vi "Resistance to temp.vi"(11 "Resistance":dbl format="%#_13p") -> (3 "Temperature":dbl)   [LabVIEW 2021]
uses:
  controls/comparison selection.ctl
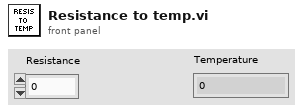
[diagram p1: front panel]
types:
  T1 = typedef "comparison selection.ctl" = enum16{"None", "in-range?", "less than?", "greater than?", "equal to?", "not equal to?", "less or equal to?", "greater or equal to?"}
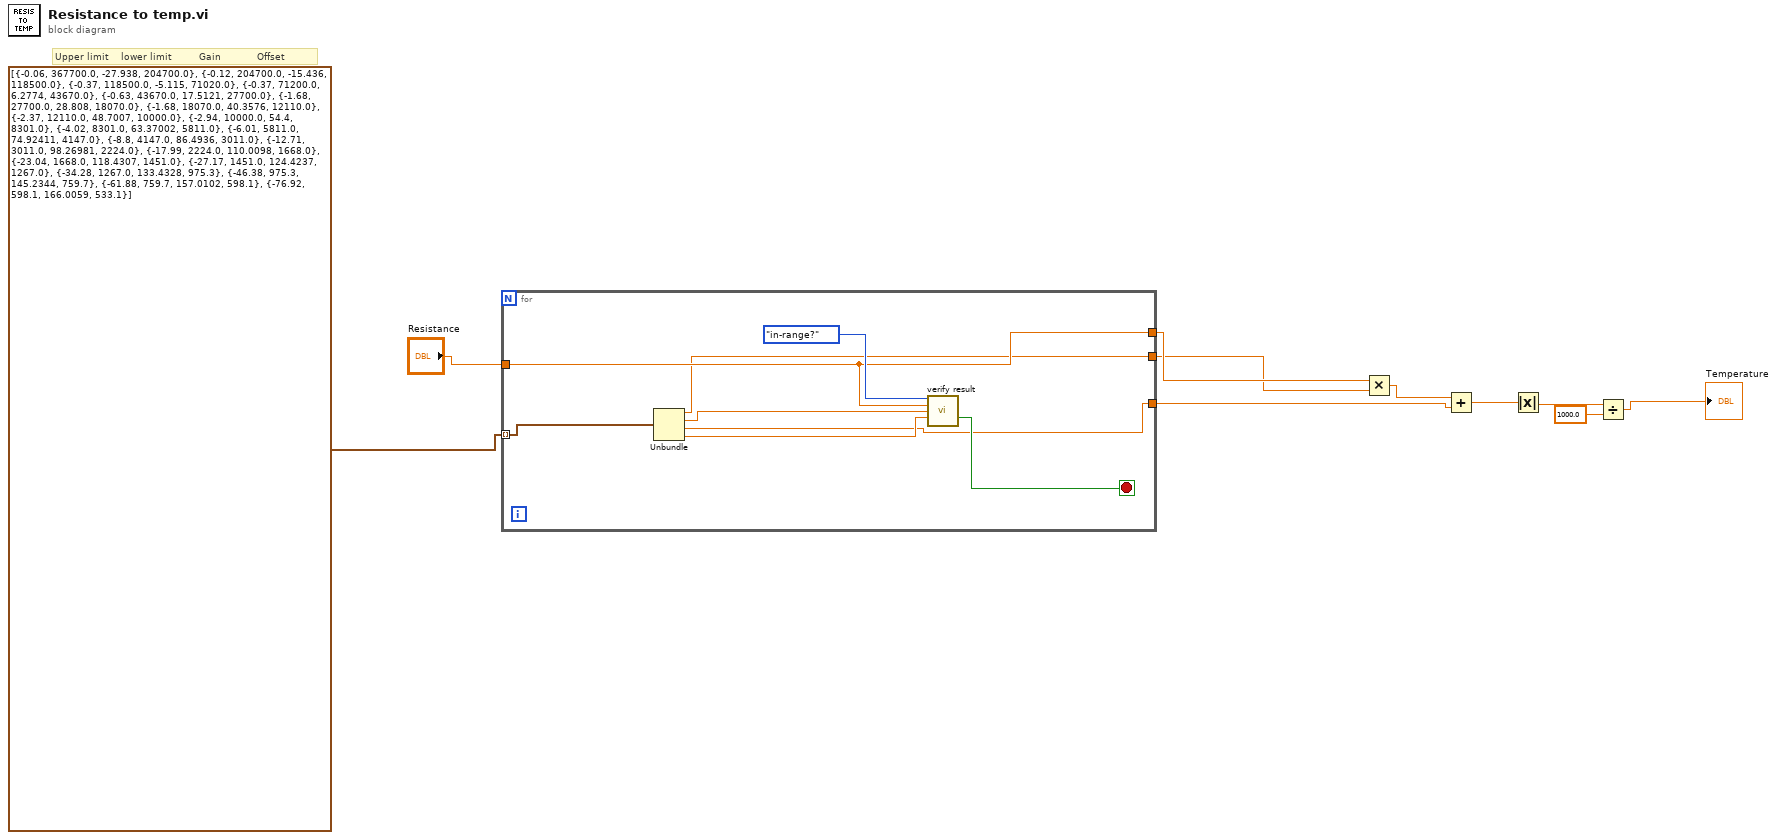
[diagram p0: block diagram]
diagram:
  # "Upper limit    lower limit         Gain            Offset"
  n1 = for {
    tunnel: cluster{dbl, dbl, dbl, dbl}[] [{-0.06, 367700.0, -27.938, 204700.0}, {-0.12, 204700.0, -15.436, 118500.0}, {-0.37, 118500.0, -5.115, 71020.0}, {-0.37, 71200.0, 6.2774, 43670.0}, {-0.63, 43670.0, 17.5121, 27700.0}, {-1.68, 27700.0, 28.808, 18070.0}, {-1.68, 18070.0, 40.3576, 12110.0}, {-2.37, 12110.0, 48.7007, 10000.0}, {-2.94, 10000.0, 54.4, 8301.0}, {-4.02, 8301.0, 63.37002, 5811.0}, {-6.01, 5811.0, 74.92411, 4147.0}, {-8.8, 4147.0, 86.4936, 3011.0}, {-12.71, 3011.0, 98.26981, 2224.0}, {-17.99, 2224.0, 110.0098, 1668.0}, {-23.04, 1668.0, 118.4307, 1451.0}, {-27.17, 1451.0, 124.4237, 1267.0}, {-34.28, 1267.0, 133.4328, 975.3}, {-46.38, 975.3, 145.2344, 759.7}, {-61.88, 759.7, 157.0102, 598.1}, {-76.92, 598.1, 166.0059, 533.1}] -> [w18] mode=indexing
    tunnel: "Resistance" -> [w15]
    tunnel: [w12] -> w5
    tunnel: [w11] -> w7
    tunnel: [w15] -> w8
    stop <- w16 stop-if-true
    n2 = Unbundle(w18) -> (w11:dbl, w14:dbl, w12:dbl, w13:dbl)
    n3 = call "verify result.vi"("comparison"=comparison_selection."in-range?", "measured data"=w15, "UL"=w14, "LL"=w13) -> ("result?"=w16:bool)  [unwired: 8 in, 3 out]
  }
  n4 = Multiply(x=w8, y=w7) -> (x*y=w6:dbl)
  n5 = Add(x=w6, y=w5) -> (x+y=w4:dbl)
  n6 = Absolute Value(x=w4) -> (abs(x)=w3:dbl)
  n7 = Divide(x=w3, y=1000.0) -> (x/y=→"Temperature":dbl)
